vi "XLIN1.7-2048SQ TE0_Begin.vi"() -> (0 "Текущий Образец №":string)   [LabVIEW 2018]
panel:
  in  "OK Button":bool
  out "Boolean 4":bool
  out "Boolean 3":bool
  in  "Образец №":string
  out "Boolean":bool
  out "Boolean 2":bool
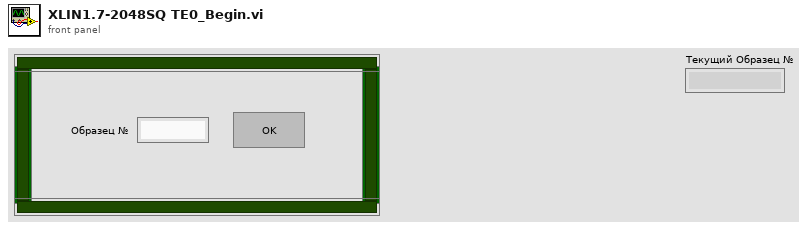
[diagram p1: front panel]
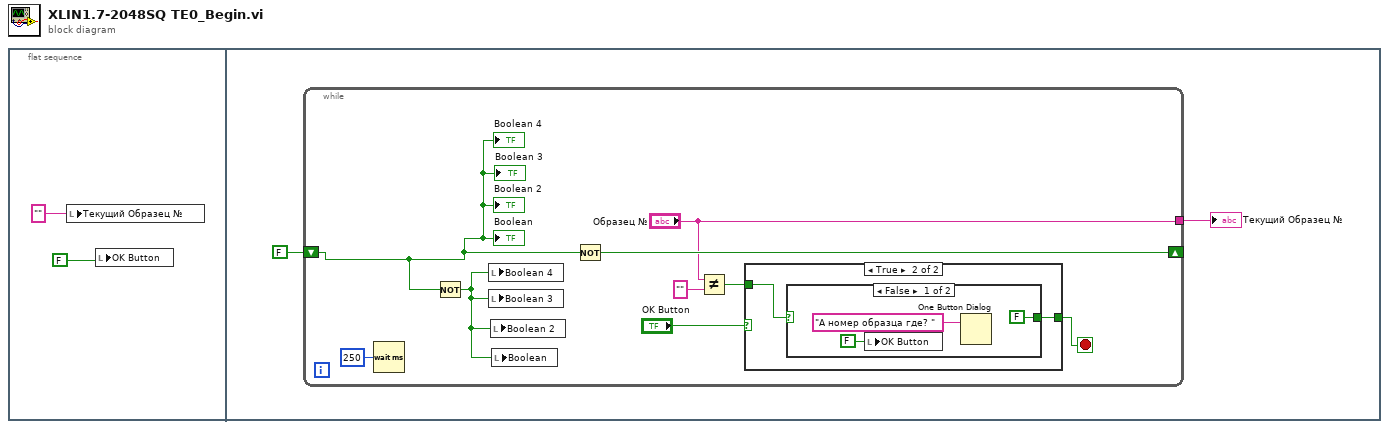
[diagram p0: block diagram]
diagram:
  n1 = flat-sequence {
    frame #0 {
      n2 = local write "Текущий Образец №"("" ("Текущий Образец № 2")) -> ()
      n3 = local write "OK Button"(FALSE ("Ввел!")) -> ()
    }
    frame #1 {
      n4 = while {
        tunnel: ["Образец №"] -> w4
        shift-right: [w12] -> _
        shift-left: FALSE -> [w11]
        stop <- w6 stop-if-true
        n5 = Wait (ms)(milliseconds to wait=u32 250) -> ()  [unwired: 1 out]
        n6 = Not(x=w11) -> (.not. x?=w10:bool)
        n7 = local write "Boolean 4"(w10) -> ()
        n8 = local write "Boolean 3"(w10) -> ()
        n9 = local write "Boolean 2"(w10) -> ()
        n10 = local write "Boolean"(w10) -> ()
        n11 = Not(x=w11) -> (.not. x?=w12:bool)
        n12 = Not Equal?(x="Образец №", y="") -> (x != y?=w7:bool)
        n13 = case shown="True" "OK Button" {
          selector: "OK Button" -> [w14 _]
          tunnel: w7 -> [_ w16]
          tunnel: [w14 w15] -> w6
          frame False {
          }
          frame True {
            n14 = case shown="False" w16 {
              selector: w16 -> [_ w20]
              tunnel: [FALSE w20] -> w15
              frame False {
                n15 = local write "OK Button"(FALSE ("OK Button")) -> ()
                n16 = One Button Dialog(message="А номер образца где? ") -> ()  [unwired: 1 in, 1 out]
              }
              frame True {
              }
            }
          }
        }
        "Boolean" <- w11
        "Boolean 2" <- w11
        "Boolean 3" <- w11
        "Boolean 4" <- w11
      }
      "Текущий Образец №" <- w4
    }
  }
